vi "Set RIO INI Key.vi"(8 "error in (no error)":errorcluster, 11 "Section Ref in":T1 format="%.0x") -> (0 "error out":errorcluster, 3 "Section Ref out":T1 format="%.0x")   [LabVIEW 2020, in "FPGA Addon Engine.lvlib"]
uses:
  FPGA Addon Engine.lvlib
  <vilib>/NI VeriStand/Custom Device API/Custom Device Item Ref.ctl
  <vilib>/Utility/config.llb/Write Key (I32).vi
  <vilib>/Utility/config.llb/NI_LVConfig.lvlib
  <vilib>/NI VeriStand/Custom Device API/Custom Device API.lvlib
  <vilib>/NI VeriStand/Custom Device API/Custom Device Target Type.ctl
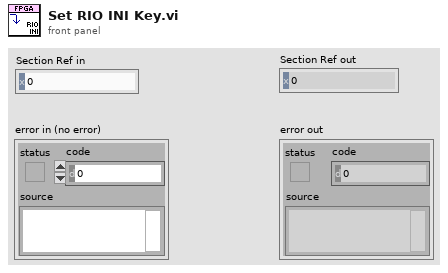
[diagram p1: front panel]
types:
  T1 = typedef "Custom Device API.lvlib/Custom Device Item Ref.ctl" = u64
  T2 = typedef "Custom Device API.lvlib/Custom Device Target Type.ctl" = enum16{"PharLap", "VxWorks", "Windows", "Linux_32_ARM", "Linux_x64"}
  T3 = typedef "NI_LVConfig.lvlib/Config Data RefNum.ctl" = refnum<k1>
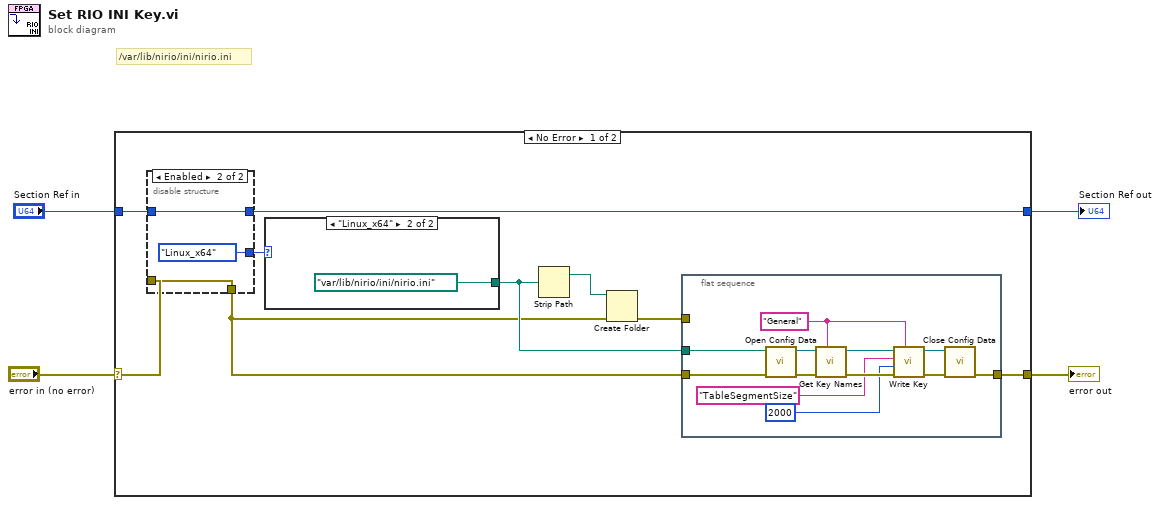
[diagram p0: block diagram]
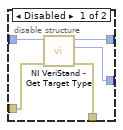
[diagram p2: hidden frame]
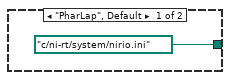
[diagram p3: hidden frame]
diagram:
  # "/var/lib/nirio/ini/nirio.ini"
  n1 = case shown="No Error" "error in (no error)" {
    selector: "error in (no error)" -> [w5 w36]
    tunnel: [w13 w36] -> w4
    tunnel: "Section Ref in" -> [w10 w37]
    tunnel: [w6 w37] -> w2
    frame No Error {
      n2 = disable-structure shown="Enabled" {
        disable-tunnel: w10 -> [w18 w20]
        disable-tunnel: [w17 Custom_Device_Target_Type."Linux_x64" ("Target Type")] -> w9
        disable-tunnel: [w16 w19] -> w7
        disable-tunnel: [w15 w20] -> w6
        disable-tunnel: w5 -> [w14 w19]
        frame Disabled {
          n3 = call <vilib>:"NI VeriStand - Get Target Type.vi"("error in (no error)"=w14, "Item Ref in"=w18) -> ("error out"=w16:errorcluster, "Target Type"=w17:T2, "Item Ref out"=w15:T1)  [unwired: 7 in]
        }
        frame Enabled {
        }
      }
      n4 = case shown="\"Linux_x64\"" w9 {
        tunnel: [path "c:/ni-rt/system/nirio.ini" ("configuration file path") path "/var/lib/nirio/ini/nirio.ini" ("configuration file path")] -> w8
        frame "PharLap", Default {
        }
        frame "Linux_x64" {
        }
      }
      n5 = Strip Path(path=w8) -> (stripped path=w12:path)  [unwired: 1 out]
      n6 = Create Folder(path (use dialog)=w12, error in=w7) -> (error out=w11:errorcluster)  [unwired: 1 in, 2 out]
      n7 = flat-sequence {
        tunnel: [w26] -> w13
        tunnel: w8 -> [w25]
        tunnel: w7 -> [w24]
        tunnel: w11 -> [_]
        frame #0 {
          w32 = "General" ("section")
          n8 = call <vilib>:"Open Config Data.vi"("error in (no error)"=w24, "configuration file path"=w25) -> ("error out"=w35:errorcluster, "refnum"=w34:T3)  [unwired: 7 in, 1 out]
          n9 = call <vilib>:"Get Key Names.vi"("section"=w32, "error in (no error)"=w35, "refnum"=w34) -> ("error out"=w31:errorcluster, "refnum out"=w33:T3)  [unwired: 5 in, 2 out]
          n10 = call-poly <vilib>:"Write Key.vi"("section"=w32, "error in (no error)"=w31, "value"=2000, "key"="TableSegmentSize", "refnum"=w33) -> ("error out"=w27:errorcluster, "refnum out"=w30:T3)  [unwired: 4 in, 1 out]
          n11 = call <vilib>:"Close Config Data.vi"("error in (no error)"=w27, "refnum"=w30) -> ("error out"=w26:errorcluster)  [unwired: 8 in, 1 out]
        }
      }
    }
    frame Error {
    }
  }
  "error out" <- w4
  "Section Ref out" <- w2
